vi "Update Status.vi"(8 "error in (no error)":errorcluster, 10 "Status":string, 11 "DiscoveryService in":refnum<class "NodeDiscovery.lvclass">) -> (0 "error out":errorcluster, 3 "DiscoveryService out":refnum<class "NodeDiscovery.lvclass">)   [LabVIEW 2020, in "Vecto.lvlib" / "NodeDiscovery.lvclass"]
uses:
  NodeDiscovery.lvclass
  NodeDiscovery.lvclass/NodeDiscovery.ctl
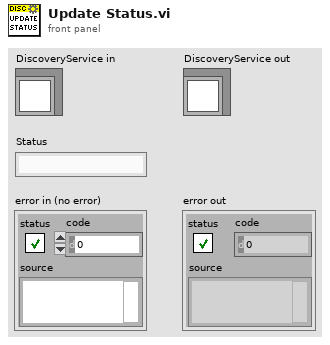
[diagram p1: front panel]
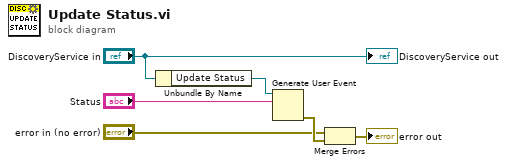
[diagram p0: block diagram]
diagram:
  n1 = Unbundle By Name("DiscoveryService in") -> ("Update Status"=w6:refnum<user-event>)
  n2 = Generate User Event(user event=w6, event data cluster="Status") -> (error out=w3:errorcluster)  [unwired: 2 in, 1 out]
  n3 = Merge Errors("error in (no error)", w3) -> (→"error out":errorcluster)
  "DiscoveryService out" <- "DiscoveryService in"
